vi "Main Page.vi"(8 "error in (no error)":errorcluster, 11 "Node Ptr":T1 format="%.0x") -> (0 "error out":errorcluster)   [LabVIEW 2023, in "Protection and Counter Addon System Explorer.lvlib"]
uses:
  Protection and Counter Addon System Explorer.lvlib
  <vilib>/NI VeriStand/Custom Device API/Custom Device Item Ref.ctl
  <vilib>/NI/NI VeriStand Hardware Resource Discovery/_Types/Filter Type.ctl
  Addon Shared/Types/986x.ctl
  Addon Shared/SubVIs/GUID Lookup.vi
  <vilib>/NI VeriStand/Custom Device API/NI VeriStand - Get Item Property.vi
  <vilib>/NI VeriStand/Custom Device API/Get Item Property (Boolean).vi
  <vilib>/NI VeriStand/Custom Device API/Get Item Property (String).vi
  <vilib>/NI VeriStand/Custom Device API/Get Item Property (Dependent File).vi
  <vilib>/NI/NI VeriStand Advanced SysDef API/_SubVIs/SysDef.Property.Set.String.vi
  <vilib>/NI/NI VeriStand Advanced SysDef API/_SubVIs/SysDef.Property.Set.U32.vi
  <vilib>/NI VeriStand/Custom Device API/Custom Device API.lvlib
  <vilib>/NI/NI VeriStand Hardware Resource Discovery/NIVS Hardware Discovery.lvlib
  Addon Shared/Protection and Counter Addon Shared.lvlib
  <vilib>/NI/NI VeriStand Advanced SysDef API/SysDef API/Advanced System Definition.lvlib
panel:
  in  "Header":cluster{"Section Name":string}={"Section Name"="Addon Settings"}
  in  "Tab Control":enum32{"Main Setting", "FPGA Settings"}(tab)
  in  "FD ISO Mode":u32(ring) items=["ISO", "Non ISO", "ISO Legacy"]
  in  "Description":string
  in  "Name":string
  out "Version":string
  in  "Port":string
  in  "CAN Browse":bool
  out "XNET Database":refnum<k21>
  out "XNET Cluster":refnum<k21>
  out "I/O Mode":u32(ring) items=["CAN 2.0", "CAN FD", "CAN FD+BRS"]
  in  "Baud Rate":u64
  in  "Termination":enum16{"Off", "On"}(ring)
  in  "FD Baud Rate":u64
  in  "Use Legacy":bool
  in  "Loop Priority":i32=100 format="%.0p"
  in  "Reselect XNET Database":bool
  in  "Enable Bitfile":bool
  in  "Bitfile Path":path
  in  "RIO Device":string
  in  "RIO Browse":bool
  in  "SHDocVw.IWebBrowser2":refnum<k7>(container)
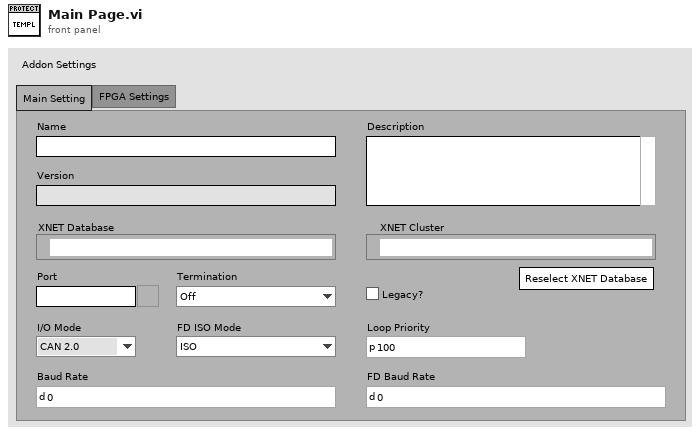
[diagram p1: front panel]
types:
  T1 = typedef "Custom Device API.lvlib/Custom Device Item Ref.ctl" = u64
  T2 = typedef "Protection and Counter Addon Shared.lvlib/986x.ctl" = cluster{"Enable":bool, "RIO Device":string, "Bitfile":path}
  T3 = typedef "Protection and Counter Addon Shared.lvlib/XNET Settings.ctl" = cluster{"Database":refnum<k21>, "Cluster":refnum<k21>, "Port":string, "Baud rate [Bd]":u64, "Termination":u32, "CAN I/O Mode":u32, "FD Baud rate [Bd]":u64, "Priority":i32, "Use Legacy":bool, "FD ISO Mode":u32}
  T4 = typedef "Custom Device API.lvlib/Custom Device Item Info.ctl" = cluster{"Name":string, "Is Channel":bool, "GUID":string, "Is Waveform":bool}
  T5 = typedef "NIVS Hardware Discovery.lvlib/Filter Type.ctl" = enum16{"Device Category", "Product Name", "Ethernet", "XNET", "VISA", "FPGA", "EtherCAT Master", "DAQmx", "GPIB", "Serial"}
  T6 = typedef "Custom Device API.lvlib/Custom Device Commands.ctl" = enum16{"Default", "Item renamed", "Shutdown", "Dynamic button pressed"}
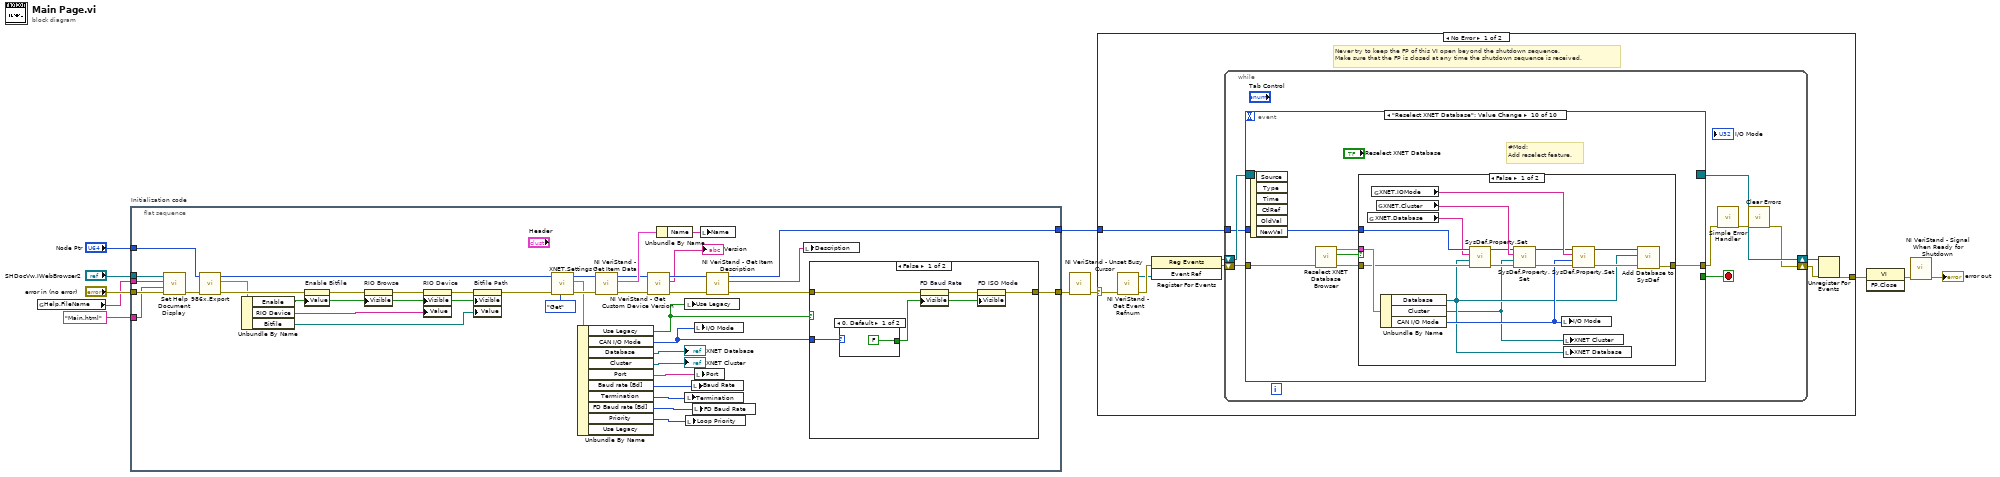
[diagram p0: block diagram]
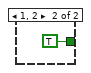
[diagram p2: hidden frame]
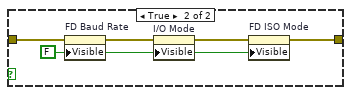
[diagram p3: hidden frame]
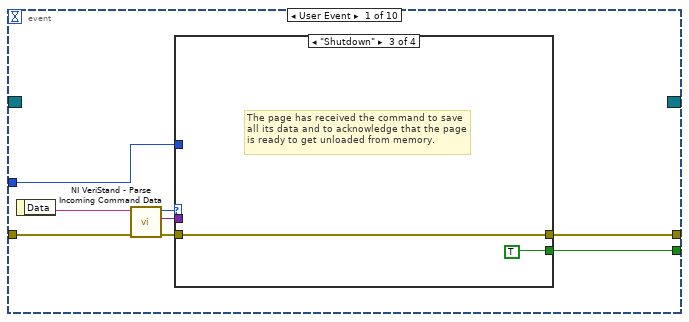
[diagram p4: hidden frame]
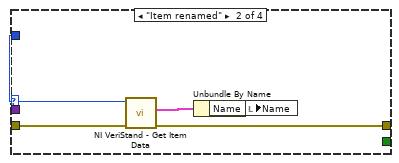
[diagram p6: hidden frame]
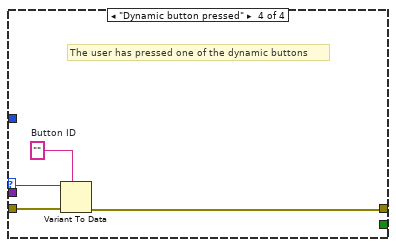
[diagram p7: hidden frame]
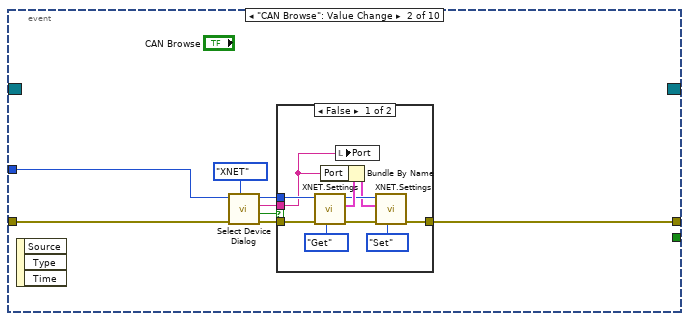
[diagram p8: hidden frame]
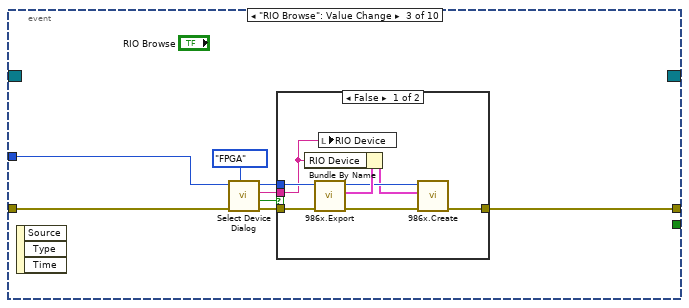
[diagram p10: hidden frame]
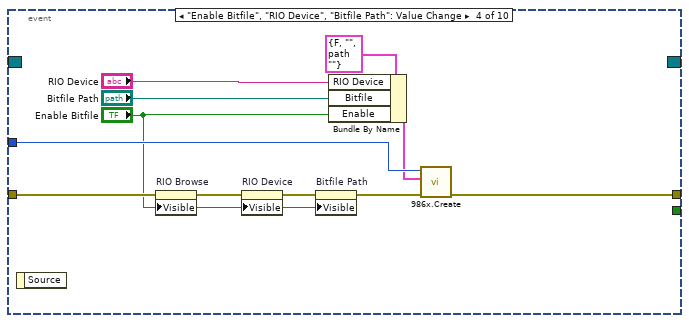
[diagram p12: hidden frame]
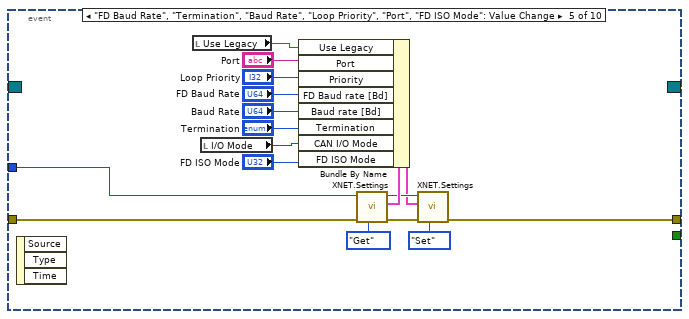
[diagram p13: hidden frame]
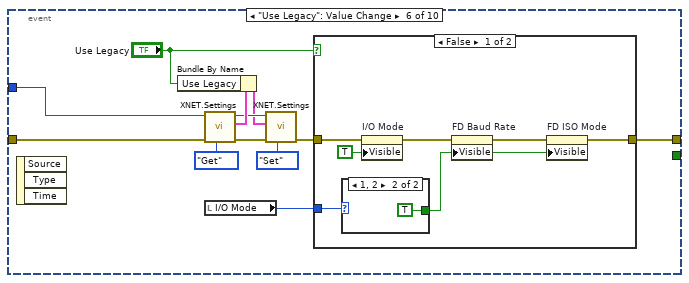
[diagram p14: hidden frame]
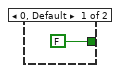
[diagram p15: hidden frame]
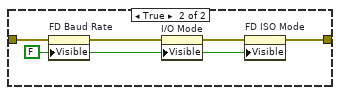
[diagram p16: hidden frame]
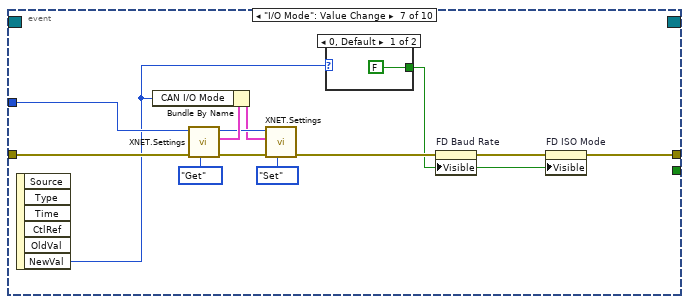
[diagram p17: hidden frame]
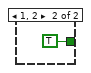
[diagram p18: hidden frame]
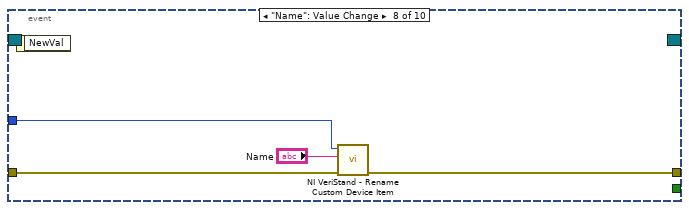
[diagram p19: hidden frame]
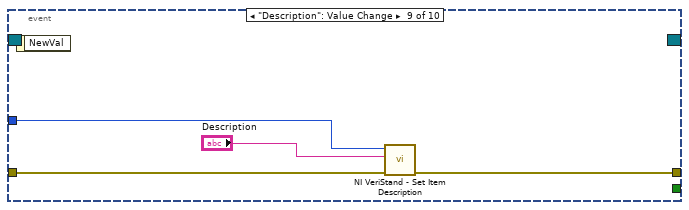
[diagram p20: hidden frame]
diagram:
  n1 = global read "GUID Lookup.vi" "Help.FileName"() -> (w1:string)
  n2 = flat-sequence "Initialization code" {
    tunnel: "error in (no error)" -> [w49]
    tunnel: "Node Ptr" -> [w30]
    tunnel: [w33] -> w7
    tunnel: [w15] -> w4
    tunnel: "SHDocVw.IWebBrowser2" -> [w48]
    tunnel: w1 -> [w47]
    tunnel: "Main.html" ("HTML File") -> [w46]
    frame #0 {
      n3 = call "Set Help Document Display.vi"("error in (no error)"=w49, "HTML File"=w46, "Main CHM File"=w47, "SHDocVw.IWebBrowser2"=w48) -> ("error out"=w31:errorcluster)  [unwired: 7 in]
      n4 = call "986x.Export.vi"("error in (no error)"=w31, "Device Item Ref in"=w30) -> ("error out"=w25:errorcluster, "986x Support"=w23:T2, "Item Ref out"=w29:T1)  [unwired: 7 in]
      n5 = Unbundle By Name(w23) -> ("Enable"=w22:bool, "RIO Device"=w21:string, "Bitfile"=w20:path)
      n6 = property on="Enable Bitfile" class="Bool (strict)"(error in=w25, "Value"=w22) -> (error out=w28:errorcluster)  [unwired: 1 in, 1 out]
      n7 = property on="RIO Browse" class="Bool"(error in=w28, "Visible"=w22) -> (error out=w27:errorcluster)  [unwired: 1 in, 1 out]
      n8 = property on="RIO Device" class="Str"(error in=w27, "Visible"=w22, "Value"=w21) -> (error out=w26:errorcluster)  [unwired: 1 in, 1 out]
      n9 = property on="Bitfile Path" class="Path"(error in=w26, "Visible"=w22, "Value"=w20) -> (error out=w24:errorcluster)  [unwired: 1 in, 1 out]
      n10 = call "XNET.Settings.vi"("Action"=enum8{"Get", "Set"}."Get", "error in (no error)"=w24, "Parent Ref in"=w29) -> ("error out"=w45:errorcluster, "XNET Settings"=w42:T3, "Item Ref out"=w44:T1)  [unwired: 6 in]
      n11 = Unbundle By Name(w42) -> ("Use Legacy"=w34:bool, "CAN I/O Mode"=w32:u32, "Database"=→"XNET Database":refnum<k21>, "Cluster"=→"XNET Cluster":refnum<k21>, "Port"=w39:string, "Baud rate [Bd]"=w38:u64, "Termination"=w37:u32, "FD Baud rate [Bd]"=w36:u64, "Priority"=w35:i32)  [unwired: 1 out]
      n12 = call <vilib>:"NI VeriStand - Get Item Data.vi"("error in (no error)"=w45, "Item Ref in"=w44) -> ("error out"=w19:errorcluster, "Item Info"=w51:T4, "Item Ref out"=w18:T1)  [unwired: 7 out]
      n13 = call <vilib>:"NI VeriStand - Get Custom Device Version.vi"("error in (no error)"=w19, "Device Ref in"=w18) -> ("error out"=w14:errorcluster, "Value"=→"Version":string, "Device Ref out"=w17:T1)  [unwired: 7 in]
      n14 = Unbundle By Name(w51) -> ("Name"=w50:string)
      n15 = local write "Use Legacy"(w34) -> ()
      n16 = local write "Termination"(w37) -> ()
      n17 = local write "Loop Priority"(w35) -> ()
      n18 = local write "Baud Rate"(w38) -> ()
      n19 = local write "FD Baud Rate"(w36) -> ()
      n20 = local write "I/O Mode"(w32) -> ()
      n21 = local write "Port"(w39) -> ()
      n22 = local write "Name"(w50) -> ()
      n23 = call <vilib>:"NI VeriStand - Get Item Description.vi"("error in (no error)"=w14, "Item Ref in"=w17) -> ("error out"=w13:errorcluster, "Description"=w12:string, "Item Ref out"=w15:T1)  [unwired: 6 in, 1 out]
      n24 = local write "Description"(w12) -> ()
      n25 = case shown="False" w34 {
        tunnel: w13 -> [w55 w62]
        tunnel: [w53 w60] -> w33
        tunnel: w32 -> [w56 _]
        frame False {
          n26 = case shown="0, Default" w56 {
            tunnel: [FALSE TRUE] -> w52
            frame 0, Default {
            }
            frame 1, 2 {
            }
          }
          n27 = property on="FD Baud Rate" class="DigNum (strict)"(error in=w55, "Visible"=w52) -> (error out=w54:errorcluster)  [unwired: 1 in, 1 out]
          n28 = property on="FD ISO Mode" class="Ring (strict)"(error in=w54, "Visible"=w52) -> (error out=w53:errorcluster)  [unwired: 1 in, 1 out]
        }
        frame True {
          w59 = FALSE ("Visible")
          n29 = property on="FD Baud Rate" class="DigNum (strict)"(error in=w62, "Visible"=w59) -> (error out=w63:errorcluster)  [unwired: 1 in, 1 out]
          n30 = property on="I/O Mode" class="Ring (strict)"(error in=w63, "Visible"=w59) -> (error out=w61:errorcluster)  [unwired: 1 in, 1 out]
          n31 = property on="FD ISO Mode" class="Ring (strict)"(error in=w61, "Visible"=w59) -> (error out=w60:errorcluster)  [unwired: 1 in, 1 out]
        }
      }
    }
  }
  n32 = call <vilib>:"NI VeriStand - Unset Busy Cursor.vi"("error in (no error)"=w7) -> ("error out"=w6:errorcluster)  [unwired: 10 out]
  n33 = case shown="No Error" w6 {
    selector: w6 -> [w64 w239]
    tunnel: [w69 w237] -> w11
    tunnel: w4 -> [w65 _]
    frame No Error {
      # "Never try to keep the FP of this VI open beyond the shutdown sequence.\nMake sure that the FP is closed at any time the shutdown sequence is received."
      n34 = call <vilib>:"NI VeriStand - Get Event Refnum.vi"("error in (no error)"=w64) -> ("error out"=w72:errorcluster, "Event Ref"=w68:refnum<user-event>)  [unwired: 9 out]
      n35 = register-events(error in=w72, w68) -> (reference out=w66:refnum<event-registration>, error out=w67:errorcluster)  [unwired: 1 in]
      n36 = while {
        tunnel: w65 -> [w76]
        shift-right: [w73] -> w70
        shift-left: w67 -> [w79]
        shift-right: [w80] -> w71
        shift-left: w66 -> [w78]
        stop <- w77 stop-if-true
        n37 = event shown="[9] \"Reselect XNET Database\": Value Change" {
          selector: w78 -> [_ _ _ _ _ _ _ _ _ _]
          dyn-events: [_ _ _ _ _ _ _ _ _ _] -> w80
          timeout: _ -> [_ _ _ _ _ _ _ _ _ _]
          tunnel: w79 -> [w88 w103 w122 w144 w158 w170 w197 w209 w213 w219]
          tunnel: [w84 _ _ _ _ _ _ _ _ _] -> w77
          tunnel: [w83 w101 w120 w147 w157 w166 w192 w208 w212 w216] -> w75
          tunnel: w76 -> [w82 w102 w121 w142 w156 w169 w196 w207 w211 w214]
          event User Event {
            n38 = event-data() -> ("Data"=w87:string)  [unwired: 1 out]
            n39 = call <vilib>:"NI VeriStand - Parse Incoming Command Data.vi"("error in (no error)"=w88, "Incoming data"=w87) -> ("error out"=w86:errorcluster, "Outgoing data"=w81:variant, "Action"=w85:T6)  [unwired: 7 out]
            n40 = case shown="\"Shutdown\"" w85 {
              tunnel: w86 -> [w89 w94 w95 w100]
              tunnel: [_ _ TRUE _] -> w84
              tunnel: [w89 w91 w95 w97] -> w83
              tunnel: w82 -> [_ w93 _ _]
              tunnel: w81 -> [_ _ _ w99]
              frame "Default", Default {
              }
              frame "Item renamed" {
                n41 = call <vilib>:"NI VeriStand - Get Item Data.vi"("error in (no error)"=w94, "Item Ref in"=w93) -> ("error out"=w91:errorcluster, "Item Info"=w92:T4)  [unwired: 8 out]
                n42 = Unbundle By Name(w92) -> ("Name"=w90:string)
                n43 = local write "Name"(w90) -> ()
              }
              frame "Shutdown" {
                # "The page has received the command to save all its data and to acknowledge that the page is ready to get unloaded from memory."
              }
              frame "Dynamic button pressed" {
                w98 = ""  # Button ID
                # "The user has pressed one of the dynamic buttons"
                n44 = Variant To Data(error in=w100, type=w98, Variant=w99) -> (error out=w97:errorcluster)  [unwired: 1 out]
              }
            }
          }
          event "CAN Browse": Value Change {
            n45 = event-data() -> ()  [unwired: 4 out]
            n46 = call <vilib>:"Select Device Dialog.vi"("Filter Type"=Filter_Type."XNET", "error in (no error)"=w103, "Item Ref in"=w102) -> ("error out"=w107:errorcluster, "Cancelled?"=w106:bool, "Selected Alias"=w105:string, "Item Ref out"=w108:T1)  [unwired: 5 in]
            n47 = case shown="False" w106 {
              tunnel: w108 -> [w116 _]
              tunnel: [w113 w119] -> w101
              tunnel: w107 -> [w110 w119]
              tunnel: w105 -> [w109 _]
              frame False {
                n48 = call "XNET.Settings.vi"("Action"=enum8{"Get", "Set"}."Get", "error in (no error)"=w110, "Parent Ref in"=w116) -> ("error out"=w111:errorcluster, "XNET Settings"=w117:T3, "Item Ref out"=w114:T1)  [unwired: 6 in]
                n49 = Bundle By Name(cluster=w117, "Port"=w109) -> (w112:T3)
                n50 = local write "Port"(w109) -> ()
                n51 = call "XNET.Settings.vi"("Action"=enum8{"Get", "Set"}."Set", "error in (no error)"=w111, "XNET Settings"=w112, "Parent Ref in"=w114) -> ("error out"=w113:errorcluster)  [unwired: 5 in, 2 out]
              }
              frame True {
              }
            }
          }
          event "RIO Browse": Value Change {
            n52 = event-data() -> ()  [unwired: 4 out]
            n53 = call <vilib>:"Select Device Dialog.vi"("Filter Type"=Filter_Type."FPGA", "error in (no error)"=w122, "Item Ref in"=w121) -> ("error out"=w126:errorcluster, "Cancelled?"=w125:bool, "Selected Alias"=w124:string, "Item Ref out"=w127:T1)  [unwired: 5 in]
            n54 = case shown="False" w125 {
              tunnel: w127 -> [w134 _]
              tunnel: [w129 w136] -> w120
              tunnel: w126 -> [w133 w136]
              tunnel: w124 -> [w132 _]
              frame False {
                n55 = call "986x.Export.vi"("error in (no error)"=w133, "Device Item Ref in"=w134) -> ("error out"=w131:errorcluster, "986x Support"=w135:T2, "Item Ref out"=w130:T1)  [unwired: 7 in]
                n56 = Bundle By Name(cluster=w135, "RIO Device"=w132) -> (w128:T2)
                n57 = local write "RIO Device"(w132) -> ()
                n58 = call "986x.Create.vi"("error in (no error)"=w131, "986x Support"=w128, "Device Item Ref in"=w130) -> ("error out"=w129:errorcluster)  [unwired: 7 in, 1 out]
              }
              frame True {
              }
            }
          }
          event "Enable Bitfile", "RIO Device", "Bitfile Path": Value Change {
            n59 = event-data() -> ()  [unwired: 2 out]
            n60 = property on="RIO Browse" class="Bool"(error in=w144, "Visible"="Enable Bitfile") -> (error out=w145:errorcluster)  [unwired: 1 in, 1 out]
            n61 = property on="RIO Device" class="Str"(error in=w145, "Visible"="Enable Bitfile") -> (error out=w146:errorcluster)  [unwired: 1 in, 1 out]
            n62 = property on="Bitfile Path" class="Path"(error in=w146, "Visible"="Enable Bitfile") -> (error out=w143:errorcluster)  [unwired: 1 in, 1 out]
            n63 = Bundle By Name(cluster=T2 {"Enable"=FALSE, "RIO Device"="", "Bitfile"=path ""} ("986x Support"), "RIO Device"="RIO Device", "Bitfile"="Bitfile Path", "Enable"="Enable Bitfile") -> (w140:T2)
            n64 = call "986x.Create.vi"("error in (no error)"=w143, "986x Support"=w140, "Device Item Ref in"=w142) -> ("error out"=w147:errorcluster)  [unwired: 7 in, 1 out]
          }
          event "FD Baud Rate", "Termination", "Baud Rate", "Loop Priority", "Port", "FD ISO Mode": Value Change {
            n65 = event-data() -> ()  [unwired: 4 out]
            n66 = local read "Use Legacy"() -> (w150:bool)
            n67 = local read "I/O Mode"() -> (w149:u32)
            n68 = call "XNET.Settings.vi"("Action"=enum8{"Get", "Set"}."Get", "error in (no error)"=w158, "Parent Ref in"=w156) -> ("error out"=w159:errorcluster, "XNET Settings"=w163:T3, "Item Ref out"=w161:T1)  [unwired: 6 in]
            n69 = Bundle By Name(cluster=w163, "Use Legacy"=w150, "Port"="Port", "Priority"="Loop Priority", "FD Baud rate [Bd]"="FD Baud Rate", "Baud rate [Bd]"="Baud Rate", "Termination"="Termination", "CAN I/O Mode"=w149, "FD ISO Mode"="FD ISO Mode") -> (w160:T3)
            n70 = call "XNET.Settings.vi"("Action"=enum8{"Get", "Set"}."Set", "error in (no error)"=w159, "XNET Settings"=w160, "Parent Ref in"=w161) -> ("error out"=w157:errorcluster)  [unwired: 5 in, 2 out]
          }
          event "Use Legacy": Value Change {
            n71 = event-data() -> ()  [unwired: 4 out]
            n72 = call "XNET.Settings.vi"("Action"=enum8{"Get", "Set"}."Get", "error in (no error)"=w170, "Parent Ref in"=w169) -> ("error out"=w171:errorcluster, "XNET Settings"=w175:T3, "Item Ref out"=w173:T1)  [unwired: 6 in]
            n73 = Bundle By Name(cluster=w175, "Use Legacy"="Use Legacy") -> (w172:T3)
            n74 = local read "I/O Mode"() -> (w165:u32)
            n75 = call "XNET.Settings.vi"("Action"=enum8{"Get", "Set"}."Set", "error in (no error)"=w171, "XNET Settings"=w172, "Parent Ref in"=w173) -> ("error out"=w167:errorcluster)  [unwired: 5 in, 2 out]
            n76 = case shown="False" "Use Legacy" {
              tunnel: w167 -> [w182 w189]
              tunnel: [w178 w187] -> w166
              tunnel: w165 -> [w183 _]
              frame False {
                n77 = case shown="1, 2" w183 {
                  tunnel: [FALSE TRUE] -> w177
                  frame 0, Default {
                  }
                  frame 1, 2 {
                  }
                }
                n78 = property on="I/O Mode" class="Ring (strict)"(error in=w182, "Visible"=TRUE) -> (error out=w181:errorcluster)  [unwired: 1 in, 1 out]
                n79 = property on="FD Baud Rate" class="DigNum (strict)"(error in=w181, "Visible"=w177) -> (error out=w179:errorcluster)  [unwired: 1 in, 1 out]
                n80 = property on="FD ISO Mode" class="Ring (strict)"(error in=w179, "Visible"=w177) -> (error out=w178:errorcluster)  [unwired: 1 in, 1 out]
              }
              frame True {
                w186 = FALSE ("Visible")
                n81 = property on="FD Baud Rate" class="DigNum (strict)"(error in=w189, "Visible"=w186) -> (error out=w190:errorcluster)  [unwired: 1 in, 1 out]
                n82 = property on="I/O Mode" class="Ring (strict)"(error in=w190, "Visible"=w186) -> (error out=w188:errorcluster)  [unwired: 1 in, 1 out]
                n83 = property on="FD ISO Mode" class="Ring (strict)"(error in=w188, "Visible"=w186) -> (error out=w187:errorcluster)  [unwired: 1 in, 1 out]
              }
            }
          }
          event "I/O Mode": Value Change {
            n84 = event-data() -> ("NewVal"=w194:u32)  [unwired: 6 out]
            n85 = call "XNET.Settings.vi"("Action"=enum8{"Get", "Set"}."Get", "error in (no error)"=w197, "Parent Ref in"=w196) -> ("error out"=w198:errorcluster, "XNET Settings"=w202:T3, "Item Ref out"=w200:T1)  [unwired: 6 in]
            n86 = Bundle By Name(cluster=w202, "CAN I/O Mode"=w194) -> (w199:T3)
            n87 = call "XNET.Settings.vi"("Action"=enum8{"Get", "Set"}."Set", "error in (no error)"=w198, "XNET Settings"=w199, "Parent Ref in"=w200) -> ("error out"=w195:errorcluster)  [unwired: 5 in, 2 out]
            n88 = case shown="0, Default" w194 {
              tunnel: [FALSE TRUE] -> w191
              frame 0, Default {
              }
              frame 1, 2 {
              }
            }
            n89 = property on="FD Baud Rate" class="DigNum (strict)"(error in=w195, "Visible"=w191) -> (error out=w193:errorcluster)  [unwired: 1 in, 1 out]
            n90 = property on="FD ISO Mode" class="Ring (strict)"(error in=w193, "Visible"=w191) -> (error out=w192:errorcluster)  [unwired: 1 in, 1 out]
          }
          event "Name": Value Change {
            n91 = event-data() -> ()  [unwired: 2 out]
            n92 = call <vilib>:"NI VeriStand - Rename Custom Device Item.vi"("error in (no error)"=w209, "New Name"="Name", "Item Ref in"=w207) -> ("error out"=w208:errorcluster)  [unwired: 1 in, 7 out]
          }
          event "Description": Value Change {
            n93 = event-data() -> ()  [unwired: 2 out]
            n94 = call <vilib>:"NI VeriStand - Set Item Description.vi"("error in (no error)"=w213, "Description"="Description", "Item Ref in"=w211) -> ("error out"=w212:errorcluster)  [unwired: 6 in, 2 out]
          }
          event "Reselect XNET Database": Value Change {
            # "#Mod:\nAdd reselect feature."
            n95 = event-data() -> ()  [unwired: 7 out]
            n96 = call "Reselect XNET Database Browser.vi"("error in (no error)"=w219) -> ("error out"=w217:errorcluster, "Cancel Out"=w218:bool, "XNET Settings"=w215:T3)  [unwired: 8 in]
            n97 = case shown="False" w218 {
              tunnel: w217 -> [w234 w236]
              tunnel: [w223 w236] -> w216
              tunnel: w215 -> [w235 _]
              tunnel: w214 -> [w233 _]
              frame False {
                n98 = global read "GUID Lookup.vi" "XNET.Database"() -> (w232:string)
                n99 = global read "GUID Lookup.vi" "XNET.IOMode"() -> (w230:string)
                n100 = global read "GUID Lookup.vi" "XNET.Cluster"() -> (w231:string)
                n101 = Unbundle By Name(w235) -> ("Database"=w221:refnum<k21>, "Cluster"=w220:refnum<k21>, "CAN I/O Mode"=w222:u32)
                n102 = call-poly <vilib>:"SysDef.Property.Set.vi"("error in (no error)"=w234, "Value"=w221, "Property Name"=w232, "nodeID"=w233) -> ("error out"=w226:errorcluster, "nodeID out"=w227:u64)  [unwired: 6 in]
                n103 = call-poly <vilib>:"SysDef.Property.Set.vi"("error in (no error)"=w226, "Value"=w220, "Property Name"=w231, "nodeID"=w227) -> ("error out"=w229:errorcluster, "nodeID out"=w228:u64)  [unwired: 6 in]
                n104 = local write "I/O Mode"(w222) -> ()
                n105 = local write "XNET Cluster"(w220) -> ()
                n106 = local write "XNET Database"(w221) -> ()
                n107 = call-poly <vilib>:"SysDef.Property.Set.vi"("error in (no error)"=w229, "Value"=w222, "Property Name"=w230, "nodeID"=w228) -> ("error out"=w224:errorcluster, "nodeID out"=w225:u64)  [unwired: 6 in]
                n108 = call "Add Database to SysDef.vi"("error in"=w224, "DB Alias"=w221, "Item Ref in"=w225) -> ("error out"=w223:errorcluster)  [unwired: 7 in, 1 out]
              }
              frame True {
              }
            }
          }
        }
        n109 = call <vilib>:"Simple Error Handler.vi"("error in (no error)"=w75) -> ("error out"=w74:errorcluster)  [unwired: 1 in, 7 out]
        n110 = call <vilib>:"Clear Errors.vi"("error in (no error)"=w74) -> ("error out"=w73:errorcluster)  [unwired: 1 in, 5 out]
      }
      n111 = Unregister For Events(event registration refnum=w71, error in=w70) -> (error out=w69:errorcluster)
    }
    frame Error {
      n112 = call <vilib>:"Simple Error Handler.vi"("error in (no error)"=w239) -> ("error out"=w238:errorcluster)  [unwired: 1 in, 7 out]
      n113 = call <vilib>:"Clear Errors.vi"("error in (no error)"=w238) -> ("error out"=w237:errorcluster)  [unwired: 1 in, 5 out]
    }
  }
  n114 = invoke class="VI" method="FP.Close"(error in=w11) -> (error out=w10:errorcluster)  [unwired: 2 in, 2 out]
  n115 = call <vilib>:"NI VeriStand - Signal When Ready for Shutdown.vi"("error in (no error)"=w10) -> ("error out"=→"error out":errorcluster)  [unwired: 10 out]
